vi "Read.vi"(8 "error in (no error)":errorcluster, 11 "Parallax PING))) FPGA in":refnum<class "Parallax PING))) FPGA.lvclass">) -> (0 "error out":errorcluster, 1 "Timed out?":bool, 2 "Distance (m)":dbl, 3 "Parallax PING))) FPGA out":refnum<class "Parallax PING))) FPGA.lvclass">)   [LabVIEW 2013, in "Parallax PING))) FPGA.lvclass"]
doc: "Reads the distance in m."
uses:
  Parallax PING))) FPGA.lvclass
  Parallax PING))) FPGA.lvclass/Parallax PING))) FPGA.ctl
  <vilib>/rvi/interface/common/niFpgaWaitOnOcc.vi
  <vilib>/rvi/errors/niLvFpgaAdjustHostInterfaceError.vi
  <vilib>/rvi/interface/nirviReadWriteControl/nirviReadWriteControl.xnode
  NiFpgaLv.dll
  <vilib>/rvi/interface/Simulation/niFpgaSimulationCallBeginRW.vi
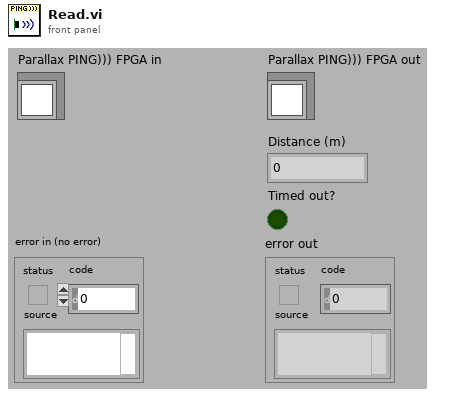
[diagram p1: front panel]
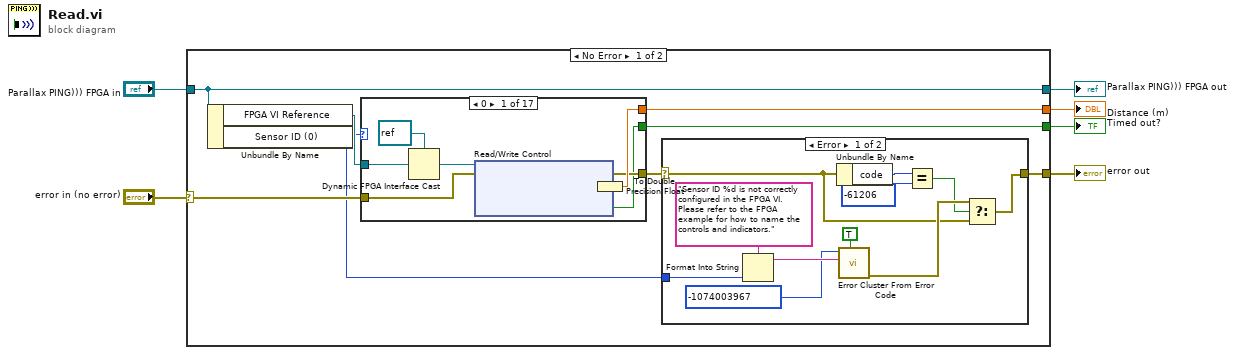
[diagram p0: block diagram]
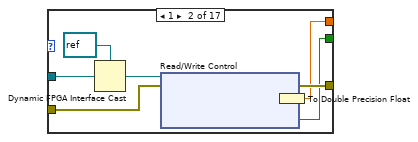
[diagram p3: hidden frame]
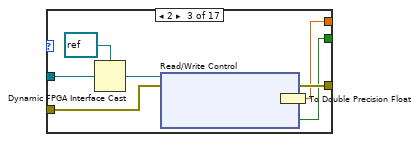
[diagram p4: hidden frame]
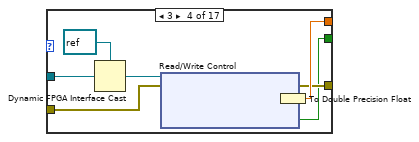
[diagram p5: hidden frame]
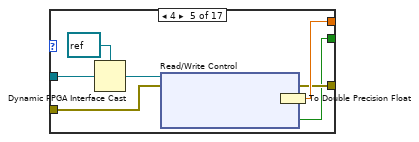
[diagram p6: hidden frame]
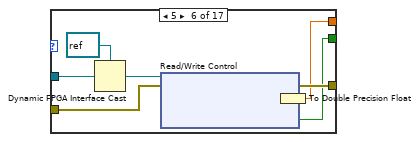
[diagram p7: hidden frame]
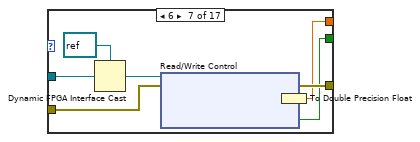
[diagram p8: hidden frame]
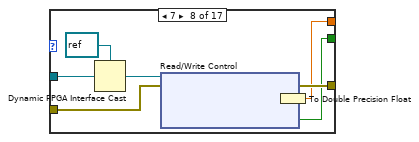
[diagram p9: hidden frame]
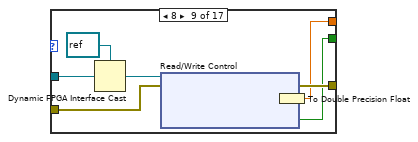
[diagram p10: hidden frame]
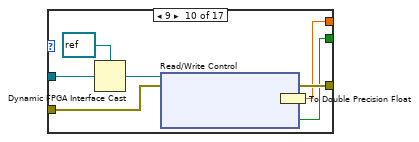
[diagram p11: hidden frame]
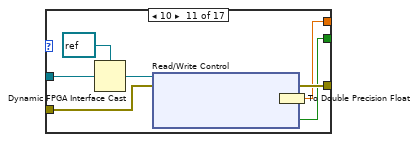
[diagram p12: hidden frame]
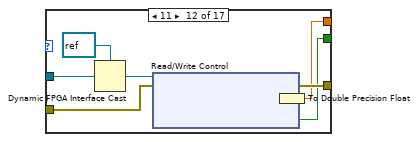
[diagram p13: hidden frame]
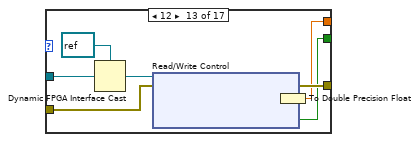
[diagram p14: hidden frame]
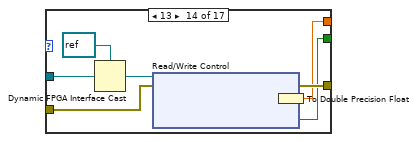
[diagram p15: hidden frame]
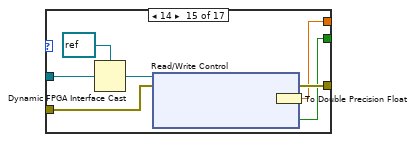
[diagram p16: hidden frame]
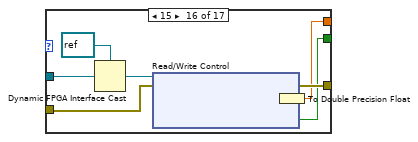
[diagram p17: hidden frame]
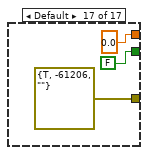
[diagram p18: hidden frame]
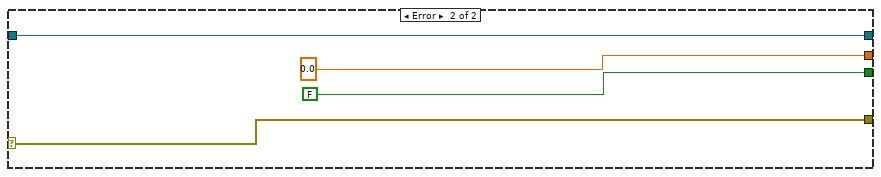
[diagram p19: hidden frame]
diagram:
  n1 = case shown="No Error" "error in (no error)" {
    selector: "error in (no error)" -> [w12 w161]
    tunnel: [w7 w161] -> w5
    tunnel: [w14 w160] -> w3
    tunnel: "Parallax PING))) FPGA in" -> [w14 w160]
    tunnel: [w11 0.0] -> w2
    tunnel: [w10 FALSE ("PING)))_0_timeout")] -> w1
    frame No Error {
      n2 = Unbundle By Name(w14) -> ("FPGA VI Reference"=w13:refnum<k20>, "Sensor ID (0)"=w8:i32)
      n3 = case shown="0" w8 {
        tunnel: w13 -> [w34 w41 w49 w57 w65 w73 w81 w89 w97 w105 w113 w121 w129 w137 w145 w153 _]
        tunnel: w12 -> [w32 w40 w48 w56 w64 w72 w80 w88 w96 w102 w112 w119 w126 w134 w144 w152 _]
        tunnel: [w30 w39 w47 w54 w62 w71 w79 w87 w95 w104 w111 w120 w128 w136 w143 w151 errorcluster {"status"=TRUE, "code"=-61206, "source"=""} ("error out")] -> w9
        tunnel: [w31 w38 w46 w55 w63 w70 w78 w86 w94 w103 w110 w118 w127 w135 w142 w150 0.0] -> w11
        tunnel: [w27 w35 w43 w51 w59 w67 w75 w83 w91 w99 w107 w115 w123 w131 w139 w147 FALSE ("PING)))_15_timeout")] -> w10
        frame 0 {
          n4 = Dynamic FPGA Interface Cast(Session In=refnum<k20> refnum ("FPGA VI Reference Out"), Type=w34) -> (Session Out=w33:refnum<k20>)
          n5 = xnode "Read/Write Control"("FPGA VI Reference In"=w33, "error in"=w32) -> ("error out"=w30:errorcluster, "PING)))_0_dist"=w28:fxp<+,32,8>, "PING)))_0_timeout"=w27:bool)  [unwired: 1 out]
          n6 = To Double Precision Float(number=w28) -> (double precision float=w31:dbl)
        }
        frame 1 {
          n7 = Dynamic FPGA Interface Cast(Session In=refnum<k20> refnum ("FPGA VI Reference Out"), Type=w41) -> (Session Out=w42:refnum<k20>)
          n8 = xnode "Read/Write Control"("FPGA VI Reference In"=w42, "error in"=w40) -> ("error out"=w39:errorcluster, "PING)))_1_dist"=w36:fxp<+,32,8>, "PING)))_1_timeout"=w35:bool)  [unwired: 1 out]
          n9 = To Double Precision Float(number=w36) -> (double precision float=w38:dbl)
        }
        frame 2 {
          n10 = Dynamic FPGA Interface Cast(Session In=refnum<k20> refnum ("FPGA VI Reference Out"), Type=w49) -> (Session Out=w50:refnum<k20>)
          n11 = xnode "Read/Write Control"("FPGA VI Reference In"=w50, "error in"=w48) -> ("error out"=w47:errorcluster, "PING)))_2_dist"=w44:fxp<+,32,8>, "PING)))_2_timeout"=w43:bool)  [unwired: 1 out]
          n12 = To Double Precision Float(number=w44) -> (double precision float=w46:dbl)
        }
        frame 3 {
          n13 = Dynamic FPGA Interface Cast(Session In=refnum<k20> refnum ("FPGA VI Reference Out"), Type=w57) -> (Session Out=w58:refnum<k20>)
          n14 = xnode "Read/Write Control"("FPGA VI Reference In"=w58, "error in"=w56) -> ("error out"=w54:errorcluster, "PING)))_3_dist"=w52:fxp<+,32,8>, "PING)))_3_timeout"=w51:bool)  [unwired: 1 out]
          n15 = To Double Precision Float(number=w52) -> (double precision float=w55:dbl)
        }
        frame 4 {
          n16 = Dynamic FPGA Interface Cast(Session In=refnum<k20> refnum ("FPGA VI Reference Out"), Type=w65) -> (Session Out=w66:refnum<k20>)
          n17 = xnode "Read/Write Control"("FPGA VI Reference In"=w66, "error in"=w64) -> ("error out"=w62:errorcluster, "PING)))_4_dist"=w60:fxp<+,32,8>, "PING)))_4_timeout"=w59:bool)  [unwired: 1 out]
          n18 = To Double Precision Float(number=w60) -> (double precision float=w63:dbl)
        }
        frame 5 {
          n19 = Dynamic FPGA Interface Cast(Session In=refnum<k20> refnum ("FPGA VI Reference Out"), Type=w73) -> (Session Out=w74:refnum<k20>)
          n20 = xnode "Read/Write Control"("FPGA VI Reference In"=w74, "error in"=w72) -> ("error out"=w71:errorcluster, "PING)))_5_dist"=w68:fxp<+,32,8>, "PING)))_5_timeout"=w67:bool)  [unwired: 1 out]
          n21 = To Double Precision Float(number=w68) -> (double precision float=w70:dbl)
        }
        frame 6 {
          n22 = Dynamic FPGA Interface Cast(Session In=refnum<k20> refnum ("FPGA VI Reference Out"), Type=w81) -> (Session Out=w82:refnum<k20>)
          n23 = xnode "Read/Write Control"("FPGA VI Reference In"=w82, "error in"=w80) -> ("error out"=w79:errorcluster, "PING)))_6_dist"=w76:fxp<+,32,8>, "PING)))_6_timeout"=w75:bool)  [unwired: 1 out]
          n24 = To Double Precision Float(number=w76) -> (double precision float=w78:dbl)
        }
        frame 7 {
          n25 = Dynamic FPGA Interface Cast(Session In=refnum<k20> refnum ("FPGA VI Reference Out"), Type=w89) -> (Session Out=w90:refnum<k20>)
          n26 = xnode "Read/Write Control"("FPGA VI Reference In"=w90, "error in"=w88) -> ("error out"=w87:errorcluster, "PING)))_7_dist"=w84:fxp<+,32,8>, "PING)))_7_timeout"=w83:bool)  [unwired: 1 out]
          n27 = To Double Precision Float(number=w84) -> (double precision float=w86:dbl)
        }
        frame 8 {
          n28 = Dynamic FPGA Interface Cast(Session In=refnum<k20> refnum ("FPGA VI Reference Out"), Type=w97) -> (Session Out=w98:refnum<k20>)
          n29 = xnode "Read/Write Control"("FPGA VI Reference In"=w98, "error in"=w96) -> ("error out"=w95:errorcluster, "PING)))_8_dist"=w92:fxp<+,32,8>, "PING)))_8_timeout"=w91:bool)  [unwired: 1 out]
          n30 = To Double Precision Float(number=w92) -> (double precision float=w94:dbl)
        }
        frame 9 {
          n31 = Dynamic FPGA Interface Cast(Session In=refnum<k20> refnum ("FPGA VI Reference Out"), Type=w105) -> (Session Out=w106:refnum<k20>)
          n32 = xnode "Read/Write Control"("FPGA VI Reference In"=w106, "error in"=w102) -> ("error out"=w104:errorcluster, "PING)))_9_dist"=w100:fxp<+,32,8>, "PING)))_9_timeout"=w99:bool)  [unwired: 1 out]
          n33 = To Double Precision Float(number=w100) -> (double precision float=w103:dbl)
        }
        frame 10 {
          n34 = Dynamic FPGA Interface Cast(Session In=refnum<k20> refnum ("FPGA VI Reference Out"), Type=w113) -> (Session Out=w114:refnum<k20>)
          n35 = xnode "Read/Write Control"("FPGA VI Reference In"=w114, "error in"=w112) -> ("error out"=w111:errorcluster, "PING)))_10_dist"=w108:fxp<+,32,8>, "PING)))_10_timeout"=w107:bool)  [unwired: 1 out]
          n36 = To Double Precision Float(number=w108) -> (double precision float=w110:dbl)
        }
        frame 11 {
          n37 = Dynamic FPGA Interface Cast(Session In=refnum<k20> refnum ("FPGA VI Reference Out"), Type=w121) -> (Session Out=w122:refnum<k20>)
          n38 = xnode "Read/Write Control"("FPGA VI Reference In"=w122, "error in"=w119) -> ("error out"=w120:errorcluster, "PING)))_11_dist"=w116:fxp<+,32,8>, "PING)))_11_timeout"=w115:bool)  [unwired: 1 out]
          n39 = To Double Precision Float(number=w116) -> (double precision float=w118:dbl)
        }
        frame 12 {
          n40 = Dynamic FPGA Interface Cast(Session In=refnum<k20> refnum ("FPGA VI Reference Out"), Type=w129) -> (Session Out=w130:refnum<k20>)
          n41 = xnode "Read/Write Control"("FPGA VI Reference In"=w130, "error in"=w126) -> ("error out"=w128:errorcluster, "PING)))_12_dist"=w124:fxp<+,32,8>, "PING)))_12_timeout"=w123:bool)  [unwired: 1 out]
          n42 = To Double Precision Float(number=w124) -> (double precision float=w127:dbl)
        }
        frame 13 {
          n43 = Dynamic FPGA Interface Cast(Session In=refnum<k20> refnum ("FPGA VI Reference Out"), Type=w137) -> (Session Out=w138:refnum<k20>)
          n44 = xnode "Read/Write Control"("FPGA VI Reference In"=w138, "error in"=w134) -> ("error out"=w136:errorcluster, "PING)))_13_dist"=w132:fxp<+,32,8>, "PING)))_13_timeout"=w131:bool)  [unwired: 1 out]
          n45 = To Double Precision Float(number=w132) -> (double precision float=w135:dbl)
        }
        frame 14 {
          n46 = Dynamic FPGA Interface Cast(Session In=refnum<k20> refnum ("FPGA VI Reference Out"), Type=w145) -> (Session Out=w146:refnum<k20>)
          n47 = xnode "Read/Write Control"("FPGA VI Reference In"=w146, "error in"=w144) -> ("error out"=w143:errorcluster, "PING)))_14_dist"=w140:fxp<+,32,8>, "PING)))_14_timeout"=w139:bool)  [unwired: 1 out]
          n48 = To Double Precision Float(number=w140) -> (double precision float=w142:dbl)
        }
        frame 15 {
          n49 = Dynamic FPGA Interface Cast(Session In=refnum<k20> refnum ("FPGA VI Reference Out"), Type=w153) -> (Session Out=w154:refnum<k20>)
          n50 = xnode "Read/Write Control"("FPGA VI Reference In"=w154, "error in"=w152) -> ("error out"=w151:errorcluster, "PING)))_15_dist"=w148:fxp<+,32,8>, "PING)))_15_timeout"=w147:bool)  [unwired: 1 out]
          n51 = To Double Precision Float(number=w148) -> (double precision float=w150:dbl)
        }
        frame Default {
        }
      }
      n52 = case shown="Error" w9 {
        selector: w9 -> [w15 w26]
        tunnel: w8 -> [w18 _]
        tunnel: [w17 w26] -> w7
        frame Error {
          n53 = Format Into String(format string="Sensor ID %d is not correctly configured in the FPGA VI. Please refer to the FPGA example for how to name the controls and indicators." ("Source (VI Name)"), w18) -> (resulting string=w22:string)  [unwired: 2 in, 1 out]
          n54 = Unbundle By Name(w15) -> ("code"=w23:i32)
          n55 = call <vilib>:"Error Cluster From Error Code.vi"("show call chain? (False)"=TRUE, "error message (\"\")"=w22, "error code (0)"=-1074003967 ("Code")) -> ("error out"=w25:errorcluster)  [unwired: 6 in]
          n56 = Equal?(x=w23, y=-61206) -> (x = y?=w24:bool)
          n57 = Select(t=w25, s=w24, f=w15) -> (s? t:f=w17:errorcluster)
        }
        frame No Error {
        }
      }
    }
    frame Error {
    }
  }
  "error out" <- w5
  "Parallax PING))) FPGA out" <- w3
  "Distance (m)" <- w2
  "Timed out?" <- w1
